vi "Set.vi"(0 "VISA resource name":refnum<visa-resource-name>, 1 "Local Lockout (0:1)":u32, 2 "ATTN (0:1)":u32, 3 "Run/Stop (1:0)":u32, 5 "Wavelength (nnnn)":dbl[unit], 6 "AVG (1:3)":u32, 9 "Range (0-Auto,1:8)":u32, 10 "Units (1:4)":u32, 11 "error in (no error)":errorcluster, 12 "Backlight (0:2)":u32, 13 "Beeper (0:1)":u32, 14 "Zero (0:1)":u32) -> (4 "VISA resource name out":refnum<visa-resource-name>, 15 "error out":errorcluster)   [LabVIEW 2009]
doc: "Sets 1830-C options in succession."
uses:
  Newport 1830-C/Newport 1830-C.lvlib
panel:
  in  "milliseconds to wait":u32=100
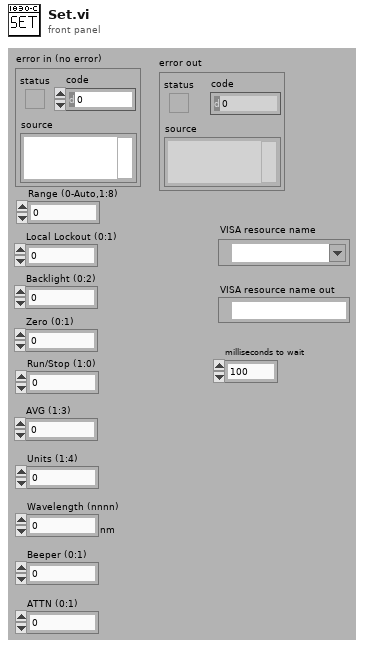
[diagram p1: front panel]
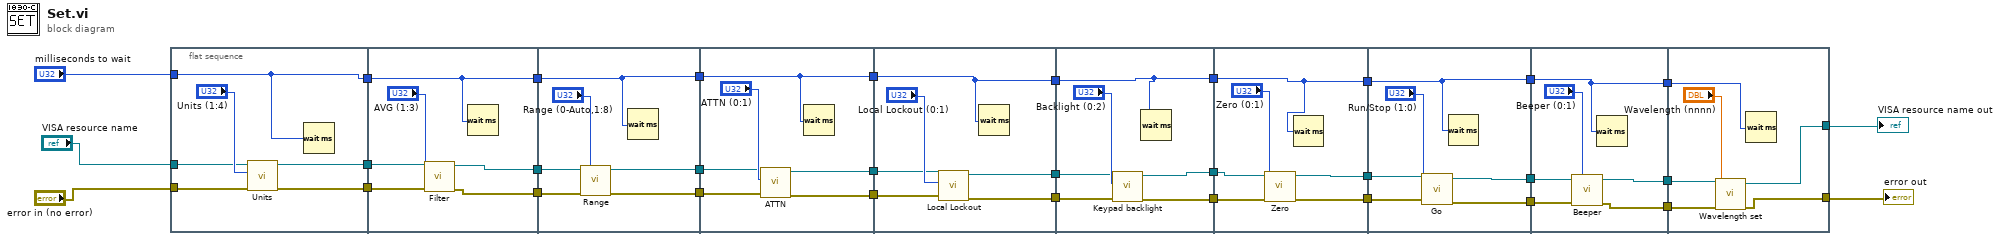
[diagram p0: block diagram]
diagram:
  n1 = flat-sequence {
    tunnel: "VISA resource name" -> [w37]
    tunnel: [w36] -> w31
    tunnel: "error in (no error)" -> [w35]
    tunnel: [w34] -> w20
    tunnel: "milliseconds to wait" -> [w34]
    tunnel: [w33] -> w9
    tunnel: w31 -> [w43]
    tunnel: [w42] -> w29
    tunnel: w20 -> [w41]
    tunnel: [w41] -> w19
    tunnel: w9 -> [w40]
    tunnel: [w39] -> w8
    tunnel: w29 -> [w49]
    tunnel: [w48] -> w28
    tunnel: w19 -> [w47]
    tunnel: [w47] -> w18
    tunnel: w8 -> [w46]
    tunnel: [w45] -> w7
    tunnel: w28 -> [w55]
    tunnel: [w54] -> w27
    tunnel: w18 -> [w53]
    tunnel: [w53] -> w17
    tunnel: w7 -> [w52]
    tunnel: [w51] -> w6
    tunnel: w27 -> [w61]
    tunnel: [w60] -> w26
    tunnel: w17 -> [w59]
    tunnel: [w59] -> w16
    tunnel: w6 -> [w58]
    tunnel: [w57] -> w5
    tunnel: w26 -> [w67]
    tunnel: [w66] -> w25
    tunnel: w16 -> [w65]
    tunnel: [w65] -> w15
    tunnel: w5 -> [w64]
    tunnel: [w63] -> w4
    tunnel: w25 -> [w73]
    tunnel: [w72] -> w24
    tunnel: w15 -> [w71]
    tunnel: [w71] -> w14
    tunnel: w4 -> [w70]
    tunnel: [w69] -> w3
    tunnel: w24 -> [w79]
    tunnel: [w78] -> w23
    tunnel: w14 -> [w77]
    tunnel: [w77] -> w13
    tunnel: w3 -> [w76]
    tunnel: [w75] -> w2
    tunnel: w23 -> [w85]
    tunnel: [w84] -> w22
    tunnel: w13 -> [w83]
    tunnel: [w83] -> w12
    tunnel: w2 -> [w82]
    tunnel: [w81] -> w1
    tunnel: w22 -> [w91]
    tunnel: [w90] -> w21
    tunnel: w12 -> [w89]
    tunnel: [w88] -> w10
    tunnel: w1 -> [w87]
    frame #0 {
      n2 = call "Units.vi"("error in (no error)"=w35, "n (0)"="Units (1:4)", "VISA resource name"=w37) -> ("error out"=w33:errorcluster, "VISA resource name out"=w36:refnum<visa-resource-name>)  [unwired: 7 in]
      n3 = Wait (ms)(milliseconds to wait=w34) -> ()  [unwired: 1 out]
    }
    frame #1 {
      n4 = call "Filter.vi"("error in (no error)"=w40, "Filter"="AVG (1:3)", "VISA resource name"=w43) -> ("error out"=w39:errorcluster, "VISA resource name out"=w42:refnum<visa-resource-name>)  [unwired: 7 in]
      n5 = Wait (ms)(milliseconds to wait=w41) -> ()  [unwired: 1 out]
    }
    frame #2 {
      n6 = call "Range.vi"("error in (no error)"=w46, "n (0)"="Range (0-Auto,1:8)", "VISA resource name"=w49) -> ("error out"=w45:errorcluster, "VISA resource name out"=w48:refnum<visa-resource-name>)  [unwired: 7 in]
      n7 = Wait (ms)(milliseconds to wait=w47) -> ()  [unwired: 1 out]
    }
    frame #3 {
      n8 = call "ATTN.vi"("error in (no error)"=w52, "Attn"="ATTN (0:1)", "VISA resource name"=w55) -> ("error out"=w51:errorcluster, "VISA resource name out"=w54:refnum<visa-resource-name>)  [unwired: 7 in]
      n9 = Wait (ms)(milliseconds to wait=w53) -> ()  [unwired: 1 out]
    }
    frame #4 {
      n10 = call "Local Lockout.vi"("error in (no error)"=w58, "n (0)"="Local Lockout (0:1)", "VISA resource name"=w61) -> ("error out"=w57:errorcluster, "VISA resource name out"=w60:refnum<visa-resource-name>)  [unwired: 7 in]
      n11 = Wait (ms)(milliseconds to wait=w59) -> ()  [unwired: 1 out]
    }
    frame #5 {
      n12 = call "Keypad backlight.vi"("error in (no error)"=w64, "BKLT"="Backlight (0:2)", "VISA resource name"=w67) -> ("error out"=w63:errorcluster, "VISA resource name out"=w66:refnum<visa-resource-name>)  [unwired: 7 in]
      n13 = Wait (ms)(milliseconds to wait=w65) -> ()  [unwired: 1 out]
    }
    frame #6 {
      n14 = call "Zero.vi"("error in (no error)"=w70, "n (0)"="Zero (0:1)", "VISA resource name"=w73) -> ("error out"=w69:errorcluster, "VISA resource name out"=w72:refnum<visa-resource-name>)  [unwired: 7 in]
      n15 = Wait (ms)(milliseconds to wait=w71) -> ()  [unwired: 1 out]
    }
    frame #7 {
      n16 = call "Go.vi"("error in (no error)"=w76, "n (0)"="Run/Stop (1:0)", "VISA resource name"=w79) -> ("error out"=w75:errorcluster, "VISA resource name out"=w78:refnum<visa-resource-name>)  [unwired: 7 in]
      n17 = Wait (ms)(milliseconds to wait=w77) -> ()  [unwired: 1 out]
    }
    frame #8 {
      n18 = call "Beeper.vi"("error in (no error)"=w82, "Beeper"="Beeper (0:1)", "VISA resource name"=w85) -> ("error out"=w81:errorcluster, "VISA resource name out"=w84:refnum<visa-resource-name>)  [unwired: 7 in]
      n19 = Wait (ms)(milliseconds to wait=w83) -> ()  [unwired: 1 out]
    }
    frame #9 {
      n20 = call "Wavelength set.vi"("error in (no error)"=w87, "Wavelength (nnnn)"="Wavelength (nnnn)", "VISA resource name"=w91) -> ("error out"=w88:errorcluster, "VISA resource name out"=w90:refnum<visa-resource-name>)  [unwired: 7 in]
      n21 = Wait (ms)(milliseconds to wait=w89) -> ()  [unwired: 1 out]
    }
  }
  "error out" <- w10
  "VISA resource name out" <- w21
